vi "Configure Serial Bus (Flexray - Trigger - Event).vi"(0 "VISA resource name":refnum<visa-resource-name>, 1 "Event BSS Frame ID (0)":i32, 5 "Serial Bus Name (1: Serial Bus 1)":i32(ring)=1 items=["Serial Bus 1"=1, "Serial Bus 2"=2], 9 "Event Type (0: Wake-Up)":i32(ring) items=["Wake-Up", "TSS", "FES", "DTS", "BSS"], 11 "error in (no error)":errorcluster) -> (4 "VISA resource name out":refnum<visa-resource-name>, 15 "error out":errorcluster)   [LabVIEW 2017, in "Agilent 2000 3000 X-Series.lvlib"]
doc: "Configures the Event Trigger settings of FlexRay bus. The event setting is only valid when the FlexRay trigger mode is set to Event.\n\nNote:\nThis VI is not supported by EDUX1052A/G, DSOX1202A/G, DSOX1204A/G models"
uses:
  Agilent 2000 3000 X-Series.lvlib
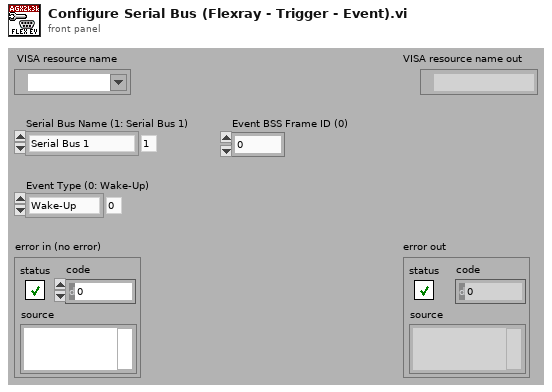
[diagram p1: front panel]
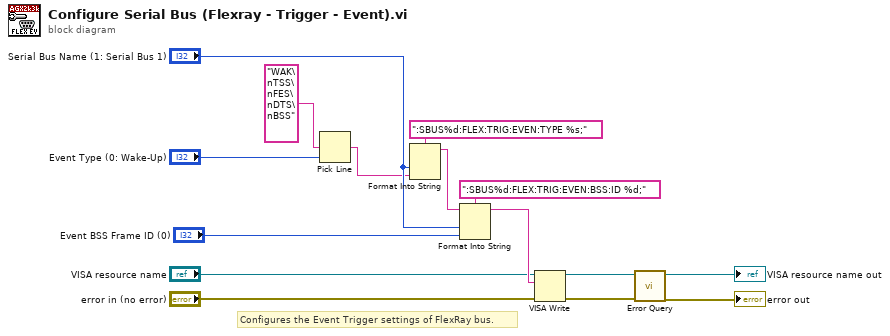
[diagram p0: block diagram]
diagram:
  # "Configures the Event Trigger settings of FlexRay bus."
  n1 = Pick Line(multi-line string="WAK\nTSS\nFES\nDTS\nBSS", line index="Event Type (0: Wake-Up)") -> (output string=w11:string)  [unwired: 1 out]
  n2 = Format Into String(format string=":SBUS%d:FLEX:TRIG:EVEN:TYPE %s;", "Serial Bus Name (1: Serial Bus 1)", w11) -> (resulting string=w10:string)  [unwired: 2 in, 1 out]
  n3 = Format Into String(format string=":SBUS%d:FLEX:TRIG:EVEN:BSS:ID %d;", initial string=w10, "Serial Bus Name (1: Serial Bus 1)", "Event BSS Frame ID (0)") -> (resulting string=w7:string)  [unwired: 1 in, 1 out]
  n4 = VISA Write(VISA resource name="VISA resource name", write buffer=w7, error in (no error)="error in (no error)") -> (VISA resource name out=w4:refnum<visa-resource-name>, error out=w3:errorcluster)  [unwired: 1 out]
  n5 = call "Error Query.vi"("error in (no error)"=w3, "VISA resource name"=w4) -> ("error out"=→"error out":errorcluster, "VISA resource name out"=→"VISA resource name out":refnum<visa-resource-name>)  [unwired: 8 out]
